vi "API Color Sensor Dev Release.vi"() -> (2 "ReleaseDev Return Value":bool)   [LabVIEW 2011, in "API ColorSensor.lvlib"]
uses:
  API ColorSensor.lvlib
  ColorSensor.dll
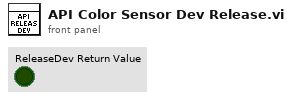
[diagram p1: front panel]
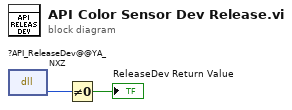
[diagram p0: block diagram]
diagram:
  n1 = dll-call lib="PTH1pabs CUsers\nAdministratorDesktop可重构机电平台项目DemoLabView基础APIColorSensor.dll" fn="?API_ReleaseDev@@YA_NXZ"() -> ("返回类型"=w2:i32)  [unwired: 3 in, 2 out]
  n2 = Not Equal To 0?(x=w2) -> (x != 0?=→"ReleaseDev Return Value":bool)
